vi "Profil X.vi"(8 "error in (no error)":errorcluster caption="entrée d'erreur (pas d'erreur)", 10 "Image in":T1(plugin-control), 11 "Acq Cam Basler en entrée":refnum<class "Acq Cam Basler.lvclass">) -> (0 "error out":errorcluster caption="sortie d'erreur", 2 "Image out":T1(plugin-control), 3 "Acq Cam Basler en sortie":refnum<class "Acq Cam Basler.lvclass">)   [LabVIEW 2023, in "Acq Cam Basler.lvclass"]
uses:
  Acq Cam Basler.lvclass
  Acq Cam Basler.lvclass/Acq Cam Basler.ctl
  <vilib>/vision/NI_Vision_Development_Module.lvlib
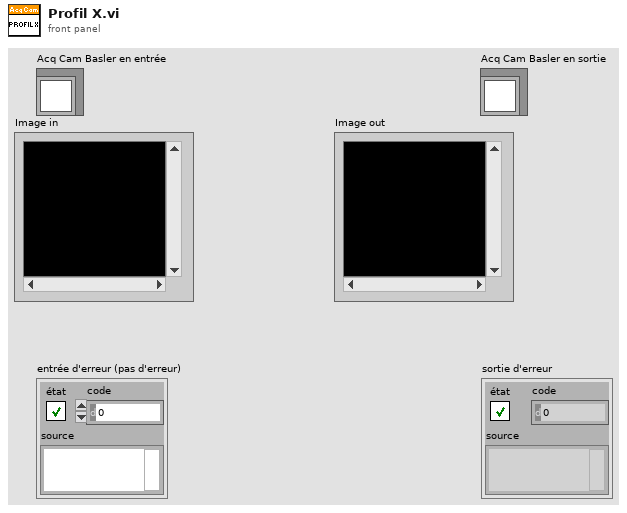
[diagram p1: front panel]
types:
  T1 = typedef "IMAQ Image.ctl" = refnum<image>
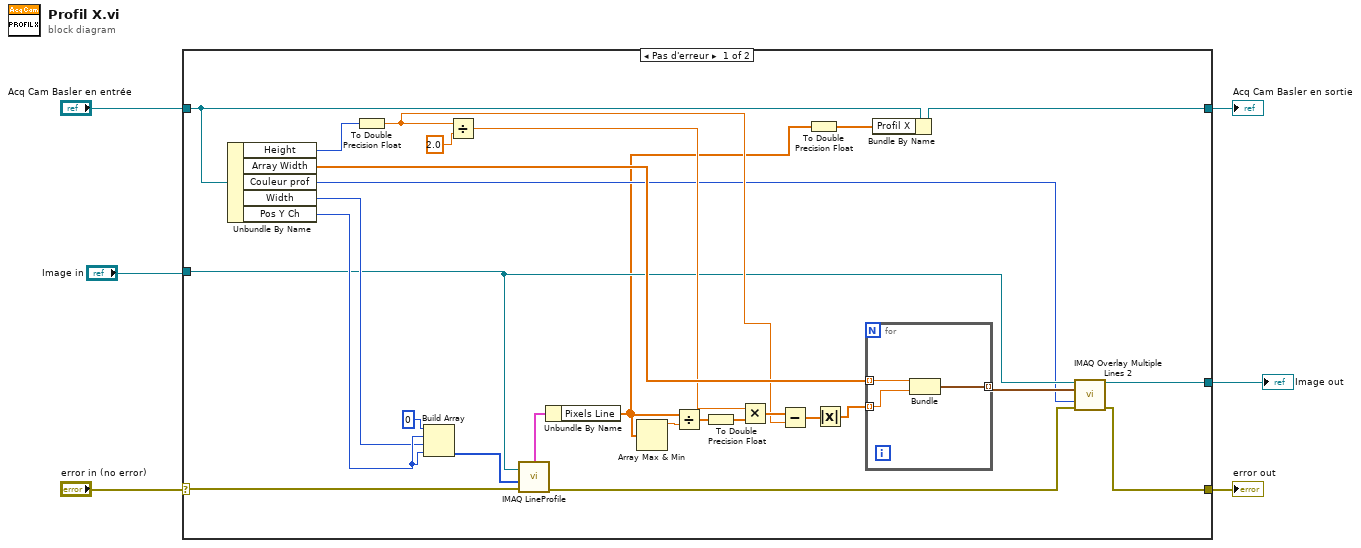
[diagram p0: block diagram]
diagram:
  n1 = case shown="Pas d'erreur" "error in (no error)" {
    selector: "error in (no error)" -> [w30 w39]
    tunnel: [w12 w39] -> w5
    tunnel: [w9 w38] -> w3
    tunnel: "Acq Cam Basler en entrée" -> [w33 w38]
    tunnel: "Image in" -> [w14 w37]
    tunnel: [w11 w37] -> w1
    frame No Error {
      n2 = Unbundle By Name(w33) -> ("Height"=w27:u32, "Array Width"=w24:dbl[], "Couleur prof"=w10:u32, "Width"=w28:u32, "Pos Y Ch"=w29:u32)
      n3 = To Double Precision Float(number=w27) -> (double precision float=w17:dbl)
      n4 = Build Array(u32 0 ("élément"), w29, w28, w29) -> (w31:u32[])
      n5 = Divide(x=w17, y=2.0) -> (x/y=w19:dbl)
      n6 = call "IMAQ LineProfile"("error in (no error)"=w30, "Line Coordinates"=w31, "Image"=w14) -> ("error out"=w13:errorcluster, "Line Graph"=w25:cluster{"x0":sgl, "dx":sgl, "Pixels Line":sgl[]})  [unwired: 2 in, 2 out]
      n7 = Unbundle By Name(w25) -> ("Pixels Line"=w8:sgl[])
      n8 = Array Max & Min(array=w8) -> (max value=w23:sgl)  [unwired: 3 out]
      n9 = Divide(x=w8, y=w23) -> (x/y=w22:sgl[])
      n10 = To Double Precision Float(number=w22) -> (double precision float=w21:dbl[])
      n11 = Multiply(x=w19, y=w21) -> (x*y=w20:dbl[])
      n12 = Subtract(x=w20, y=w17) -> (x-y=w18:dbl[])
      n13 = To Double Precision Float(number=w8) -> (double precision float=w7:dbl[])
      n14 = Absolute Value(x=w18) -> (abs(x)=w16:dbl[])
      n15 = for {
        tunnel: w24 -> [w36] mode=indexing
        tunnel: w16 -> [w35] mode=indexing
        tunnel: [w34] -> w15 mode=indexing
        n16 = Bundle("Numérique"=w36, w35) -> (w34:cluster{"Numérique":dbl, dbl})  [unwired: 1 in]
      }
      n17 = Bundle By Name(cluster=w33, "Profil X"=w7) -> (w9:refnum<class "Acq Cam Basler.lvclass">)
      n18 = call "IMAQ Overlay Multiple Lines 2"("Image"=w14, "Line End Points"=w15, "Color"=w10, "error in (no error)"=w13) -> ("Image Out"=w11:T1, "error out"=w12:errorcluster)  [unwired: 10 in]
    }
    frame Error {
    }
  }
  "error out" <- w5
  "Acq Cam Basler en sortie" <- w3
  "Image out" <- w1
